vi "deinitialize.vi"(0 "HGF_DIMEvent":refnum<class "HGF_DIMEvent.lvclass">, 5 "error in (no error)":errorcluster) -> (19 "error out":errorcluster)   [LabVIEW 2012, in "HGF_DIM.lvlib" / "HGF_DIMEvent.lvclass"]
doc: "This is a dynamic dispatch VI. It can be overwritten by childclasses to release allocated recources."
uses:
  HGF_DIMEvent.lvclass
  HGF_BaseClasses/HGF_NetworkEvent/HGF_NetworkEvent.lvclass/HGF_NetworkEvent.lvclass
  HGF_DIMEvent.lvclass/HGF_DIMEvent.ctl
  DimLVEvent/LVDimInterface/LVDimInterface.lvlib
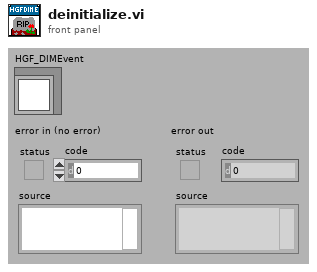
[diagram p1: front panel]
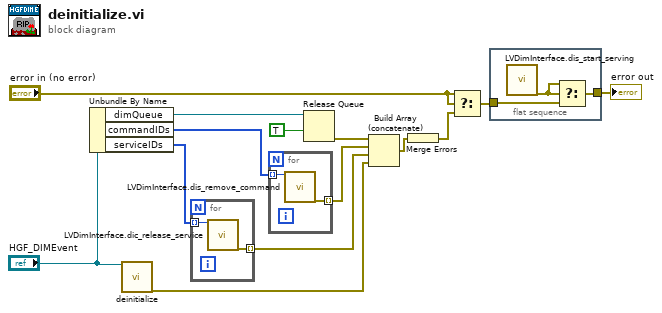
[diagram p0: block diagram]
diagram:
  n1 = Unbundle By Name("HGF_DIMEvent") -> ("dimQueue"=w12:refnum<queue>, "commandIDs"=w11:i32[], "serviceIDs"=w10:i32[])
  n2 = call-parent "deinitialize.vi"("HGF_Factory"="HGF_DIMEvent") -> ("error out"=w5:errorcluster)  [unwired: 1 in, 17 out]
  n3 = for {
    tunnel: w10 -> [w16] mode=indexing
    tunnel: [w15] -> w6 mode=indexing
    n4 = call "LVDimInterface.dic_release_service.vi"("callBackID"=w16) -> ("error out"=w15:errorcluster)  [unwired: 1 in, 17 out]
  }
  n5 = for {
    tunnel: w11 -> [w18] mode=indexing
    tunnel: [w17] -> w7 mode=indexing
    n6 = call "LVDimInterface.dis_remove_command.vi"("commandID"=w18) -> ("error out"=w17:errorcluster)  [unwired: 1 in, 17 out]
  }
  n7 = Release Queue(queue=w12, force destroy? (F)=TRUE) -> (error out=w9:errorcluster)  [unwired: 1 in, 2 out]
  n8 = Build Array (concatenate)(w9, w7, w6, w5) -> (w4:errorcluster[])
  n9 = Merge Errors(w4) -> (w3:errorcluster)
  n10 = Select(t="error in (no error)", s="error in (no error)", f=w3) -> (s? t:f=w2:errorcluster)
  n11 = flat-sequence {
    tunnel: w2 -> [w20]
    tunnel: [w19] -> w1
    frame #0 {
      n12 = call "LVDimInterface.dis_start_serving.vi"() -> ("error out"=w21:errorcluster)  [unwired: 2 in, 17 out]
      n13 = Select(t=w21, s=w21, f=w20) -> (s? t:f=w19:errorcluster)
    }
  }
  "error out" <- w1
